vi "tkrsa6100 Config Spectrum Signal Search.vi"(0 "VISA Resource Name":refnum<visa-resource-name>, 1 "Trace (1)":enum16{"1", "2", "3", "MATH", "SGRAM"}(ring), 2 "Measurement\n(SPECTRUM)":enum16{"SPECTRUM"}(ring), 5 "Set/Read\nSearch Setting (SET)":enum16{"SET", "READ"}(ring), 7 "Search Setting\n(SEARCH ON)":T2(ring), 9 "Search Criteria\n(< THRESHOLD)":T1(ring), 11 "error in (no error)":errorcluster, 12 "Threshold (0)":dbl min=-100.0 max=10000000.0 step=1e-15 format="%#.15g", 13 "Filename\n(Empty String)":string) -> (4 "dup VISA Resource Name":refnum<visa-resource-name>, 6 "Search Setting\nResponse String":string, 8 "# Fails":i32, 15 "error out":errorcluster {"code" format="%#.0f"})   [LabVIEW 2020, in "Library Instrument & Equipement.lvlib" / "Library Spectrum Analyser.lvlib"]
doc: "Prerequisites for use:\n \nThis VI is valid in the Spectrum measurement available in the General RF Measurements group.\n\nThis VI controls the following signal search functions:\nSets/reads whether the search function is on or off\nSets/reads the trace to search\nSets/reads the search criteria\nSet/reads the search threshold\nSets/reads the status of the beep on match function\nSets/reads the status of the stop acquisitions on match function\nSets/reads the status of the autosave acquisition data on match function\nSets/reads the status of the autosave trace on match function\nSets/reads the status of the autosave picture on match function\nSaves the search mask to a file\nLoads the search mask from a file\nReads the search results\n\nerror in (no error) is checked by tkrsa6100 Write/Read wError Query.vi for any pending errors.\n\nIf error in status is ERROR:\n\nerror in (no error) and VISA Resource Name are passed straight through to error out and dup VISA Resource Name of the Write/Read Drivers and returned to the calling function. No commands are processed.\n\nIf error in status is NO ERROR:\n\nBy passing SET to Set/Read Search Setting (SET) the following parameters can be written.\nPass the following selections to enumerated control Search Setting (SEARCH ON). Additional parameters to be passed are specified with each function.\n\nOne command/query is executed per VI call.\n\nSEARCH ON\nSEARCH OFF\nEnables/disables the signal search function. No further parameters necessary to be passed.\n\nSEARCH TRACE\nSelects the trace to search. Pass the trace to enumerated control Trace (1).\n\nSEARCH CRITERIA \nSelects the criteria for the signal search. Pass the selection to enumerated control Criteria (< THRESHOLD).\n\nSEARCH THRESHOLD\nSets the threshold in dBm for the search function when the criteria is set to < Threshold or >Threshold. Pass the desired threshold to numeric control Threshold (0).\n\nNote: If this function is selected when Search Criteria is set to Inside or Outside Mask error -200 \"Execution error,Scalar operation is not currently selected\" is returned.\n\nBEEP ON MATCH ON\nBEEP ON MATCH OFF\nEnables/disables the beep on match search function. No further parameters necessary to be passed.\n\nSTOP ON MATCH ON\nSTOP ON MATCH OFF\nEnables/disables the stop acquisitions on match search function. No further parameters necessary to be passed.\n\nAUTOSAVE ACQ DATA ON MATCH ON\nAUTOSAVE ACQ DATA ON MATCH OFF\nEnables/disables the autosave acquisition data on match search function. No further parameters necessary to be passed. The file is saved to the last directory used for a Load or Save As function. The filename is <base name>-<date/time stamp>.tiq. If the base name has been changed future Save As and Autosave functions will use the new base name.\n\nAUTOSAVE TRACE ON MATCH ON\nAUTOSAVE TRACE ON MATCH OFF\nEnables/disables the autosave trace data on match search function. No further parameters necessary to be passed. The file is saved to the last directory used for a Load or Save As function. The filename is <base name>-<date/time stamp>.Specan. If the base name has been changed future Save As and Autosave functions will use the new base name.\n\nAUTOSAVE PICTURE ON MATCH ON\nAUTOSAVE PICTURE ON MATCH OFF\nEnables/disables the autosave picture on match search function. No further parameters necessary to be passed. The file is saved to the last directory used for a Load or Save As function. The filename is <base name>-<date/time stamp>.png. If the base name has been changed future Save As and Autosave functions will use the new base name.\n\nSAVE SEARCH MASK TO FILE (SET)\nSet Only\nSaves the selected search mask to a .csv file. Pass the desired file path to string control Filename (Empty String).\n\nNote: Either the filename or the full file path can be specified. No quotes are necessary around the filename and no suffix is required. The instrument firmware will add the suffix as .csv. If the full file path is not specified the file will be saved to the last directory used for Save As or Open functions. This directory can be viewed by going to the Mask Editor and selecting the Load button in the UI.\n\nLOAD SEARCH MASK FROM FILE (SET)\nSet Only\nLoads the selected search mask from a .csv file. Pass the desired file path to string control Filename (Empty String).\n\nNote: Either the filename or the full file path can be specified. No quotes are necessary around the filename and no suffix is required. The instrument firmware will add the suffix as .csv. If the full file path is not specified the file will be loaded from the last directory used for Save As or Open functions. . This directory can be viewed by going to the Mask Editor and selecting the Load button in the UI.\n\nThe following parameters can be read by passing READ to enumerated control Set/Read Search Settings (SET). Pass the following values to Search Setting (SEARCH ON). The current values are returned in string indicator Search Setting Response String.\n\nSEARCH ON\nSEARCH OFF\nEither selection returns whether the signal search function is enabled or disabled. No further parameters necessary to be passed.\n\nValid Return Values:\n0 (Disabled)\n1 (Enabled)\n\nSEARCH TRACE\nReturns the current trace that is being searched. No further parameters necessary to be passed.\n\nValid Return Values:\nSpectrum: Trace 1\nSpectrum: Trace 2\nSpectrum: Trace 3\nSpectrum: Math Trace\nSpectrum: Spectrogram Trace\n\nSEARCH CRITERIA \nReturns the criteria for the signal search. No further parameters necessary to be passed.\n\nValid Return Values:\n\nLT (Less Than Threshold)\nGT (Greater Than Threshold)\nIMAS (Inside Mask)\nOMAS (Outside Mask)\n\nSEARCH THRESHOLD\nReturns the threshold in the current vertical scale units for the search function when the criteria is set to < Threshold or >Threshold. . No further parameters necessary to be passed.\n\nValid Return Value Range: -100 to 100 (dBm)\n\nNote: The valid range is dependent on the current vertical scale units setting. \n\nBEEP ON MATCH ON\nBEEP ON MATCH OFF\nReturns whether the beep on match search function is enabled or disabled. No further parameters necessary to be passed.\n\nValid Return Values:\n0 (Disabled)\n1 (Enabled)\n\nSTOP ON MATCH ON\nSTOP ON MATCH OFF\nReturns whether the stop acquisitions on match search function is enabled or disabled. No further parameters necessary to be passed.\n\nValid Return Values:\n0 (Disabled)\n1 (Enabled)\n\nAUTOSAVE ACQ DATA ON MATCH ON\nAUTOSAVE ACQ DATA ON MATCH OFF\nReturns whether the save acquisition data on match search function is enabled or disabled. No further parameters necessary to be passed.\n\nValid Return Values:\n0 (Disabled)\n1 (Enabled)\n\nAUTOSAVE TRACE ON MATCH ON\nAUTOSAVE TRACE ON MATCH OFF\nReturns whether the save trace data on match search function is enabled or disabled. No further parameters necessary to be passed.\n\nValid Return Values:\n0 (Disabled)\n1 (Enabled)\n\nAUTOSAVE PICTURE ON MATCH ON\nAUTOSAVE PICTURE ON MATCH OFF\nReturns whether the save picture on match search function is enabled or disabled. No further parameters necessary to be passed.\n\nValid Return Values:\n0 (Disabled)\n1 (Enabled)\n\nSEARCH RESULTS (READ)\nRead Only\nReturns the results from the current signal search. No further parameters necessary to be passed.\n\nThe frequency pairs portion of the search results are returned as a comma-separated list in string indicator Search Setting Response String (see notes below). If there are no failures the frequency pairs portion will be an empty string.\n\nThe number of search violations (frequency pairs) is returned in numeric indicator # Fails. If there are no failures, a 0 will be returned.\n\nNotes on Signal Search Results\n\nAll frequencies returned are in Hz.\n\nWhen either the fixed threshold or variable frequency/amplitude search mask is used the highlighted area displayed in the UI is the area that will trigger a mask violation if a signal is present inside of it.\n\nSearch results returns the number of failures and pairs of frequencies, the first being the lowest frequency that violated the mask and the second being the frequency at which the mask violation ceased.\n\nIf the displayed signal begins outside the violation area, then enters the violation area and stays within the violation area to the maximum on-screen frequency the frequencies returned are the violation frequency and the maximum on-screen frequency.\n\nIf the displayed signal begins within the violation area and then transitions out of it, the frequencies returned are the minimum on-screen frequency and the frequency at which the violation ceased.\n\nIf the entire displayed signal is in the violation area, the frequencies returned are the lowest and highest on-screen frequencies.\n\nIf the entire displayed signal is outside the violation area, the results query returns a 0.\n\nComplete Response String Format: # failures,min violation freq1,max violation freq1;min violation freq2,max violation freq2;……min violation freq(n),max violation freq(n)\n\nThe driver separates the response string at the first comma and returns # failures as an integer in numeric indicator # Fails and the remaining frequency pairs in string indicator Search Setting Response String.\n\nThe appropriate command/query string is passed to tkrsa6100 Write/Read wError Query.vi. VI Input Error Query? is set to YES by default so query SYST:ERR? is appended to the command string and the current error information is returned in cluster Error Out. \nOn completion dup VISA Resource Name, Error Out, and Search Setting Response String are returned to the calling function."
uses:
  Library Spectrum Analyser.lvlib
panel:
  # "RSA6100 Config Spectrum Signal Search Driver"
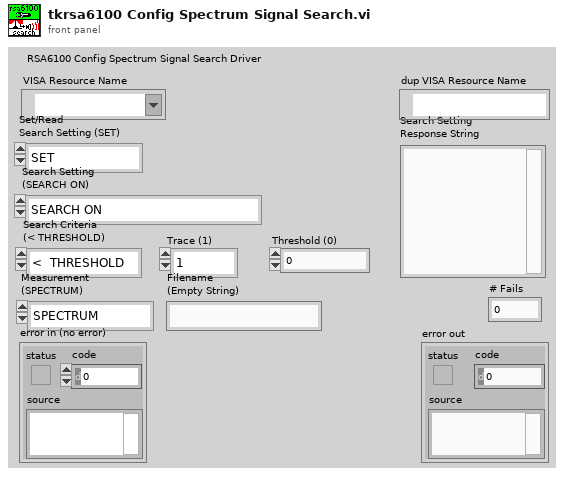
[diagram p1: front panel]
types:
  T1 = enum16{"<  THRESHOLD", "> THRESHOLD", "INSIDE MASK", "OUTSIDE MASK"}
  T2 = enum16{"SEARCH ON", "SEARCH OFF", "SEARCH TRACE", "SEARCH CRITERIA", "SEARCH THRESHOLD", "BEEP ON MATCH ON", "BEEP ON MATCH OFF", "STOP ON MATCH ON", "STOP ON MATCH OFF", "AUTOSAVE ACQ DATA ON MATCH ON", "AUTOSAVE ACQ DATA ON MATCH OFF", "AUTOSAVE TRACE ON MATCH ON", "AUTOSAVE TRACE ON MATCH OFF", "AUTOSAVE PICTURE ON MATCH ON", "AUTOSAVE PICTURE ON MATCH OFF", "SAVE SEARCH MASK TO FILE (SET)", "LOAD SEARCH MASK FROM FILE (SET)", "SEARCH RESULTS (READ)"}
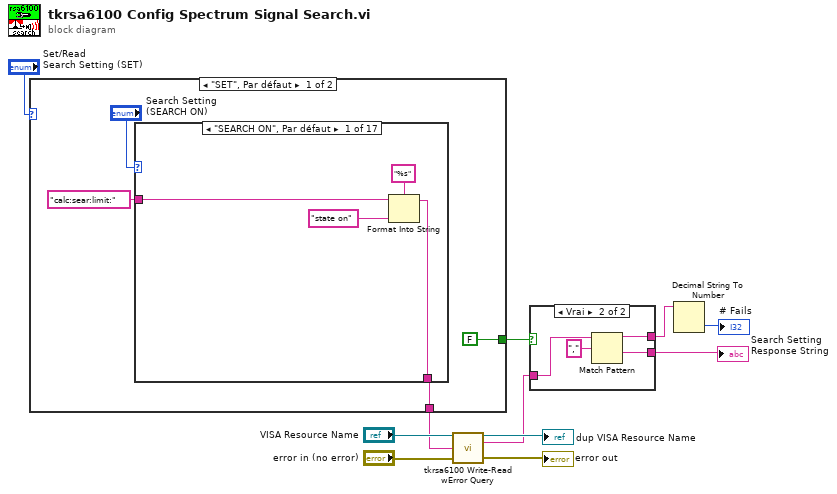
[diagram p0: block diagram]
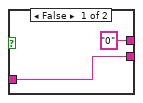
[diagram p2: hidden frame]
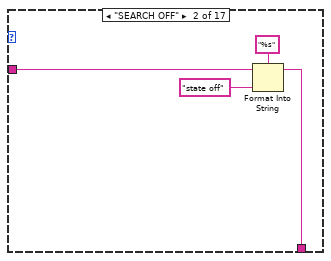
[diagram p3: hidden frame]
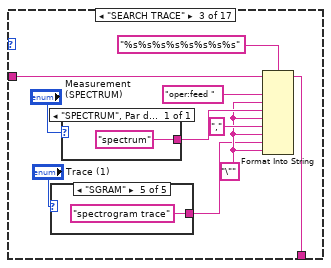
[diagram p4: hidden frame]
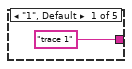
[diagram p5: hidden frame]
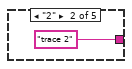
[diagram p6: hidden frame]
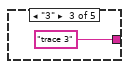
[diagram p7: hidden frame]
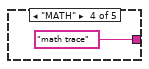
[diagram p8: hidden frame]
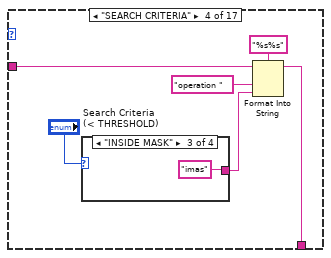
[diagram p9: hidden frame]
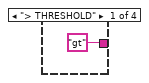
[diagram p10: hidden frame]
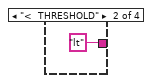
[diagram p11: hidden frame]
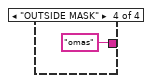
[diagram p12: hidden frame]
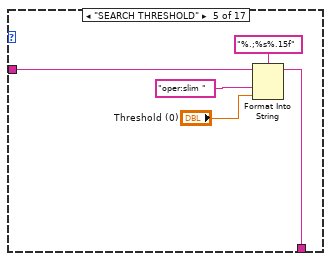
[diagram p13: hidden frame]
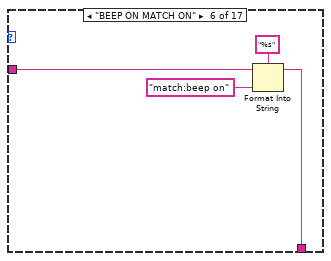
[diagram p14: hidden frame]
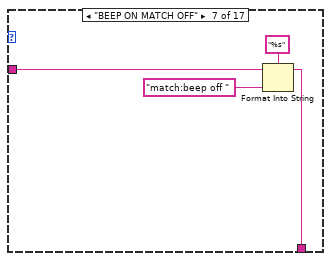
[diagram p15: hidden frame]
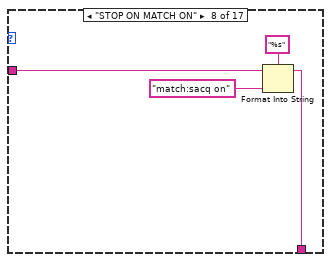
[diagram p16: hidden frame]
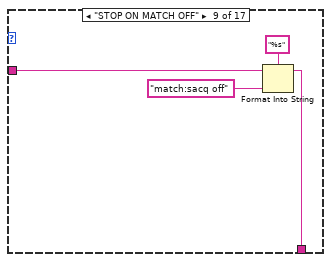
[diagram p17: hidden frame]
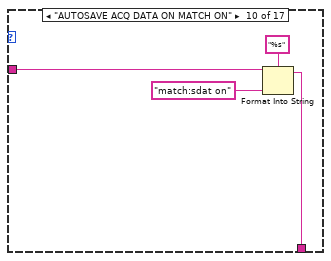
[diagram p18: hidden frame]
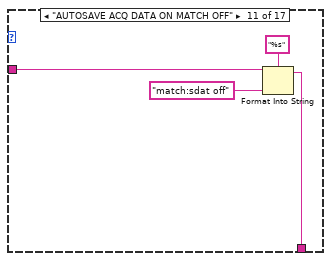
[diagram p19: hidden frame]
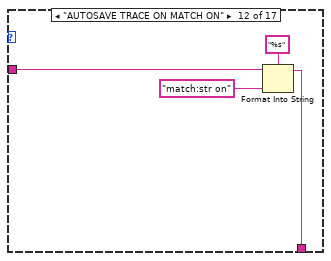
[diagram p20: hidden frame]
diagram:
  n1 = case shown="\"SET\", Par défaut" "Set/Read\nSearch Setting (SET)" {
    tunnel: [w15 w109] -> w6
    tunnel: [FALSE w107] -> w4
    frame "SET", Default {
      n2 = case shown="\"SEARCH ON\", Par défaut" "Search Setting\n(SEARCH ON)" {
        tunnel: [w18 w22 w32 w44 w53 w57 w61 w65 w69 w73 w77 w81 w85 w89 w93 w99 w105] -> w15
        tunnel: "calc:sear:limit:" ("format string") -> [w16 w21 w29 w43 w52 w56 w60 w64 w68 w71 w75 w79 w83 w87 w91 w97 w103]
        frame "SEARCH ON", Default {
          n3 = Format Into String(format string="%s", initial string=w16, "state on" ("input 1")) -> (resulting string=w18:string)  [unwired: 1 in, 1 out]
        }
        frame "SEARCH OFF" {
          n4 = Format Into String(format string="%s", initial string=w21, "state off" ("input 1")) -> (resulting string=w22:string)  [unwired: 1 in, 1 out]
        }
        frame "SEARCH TRACE" {
          w25 = "\"" ("input 1")
          n5 = case shown="\"SGRAM\"" "Trace (1)" {
            tunnel: ["trace 1" ("format string") "trace 2" ("format string") "trace 3" ("format string") "math trace" ("format string") "spectrogram trace" ("format string")] -> w24
            frame "1", Default {
            }
            frame "2" {
            }
            frame "3" {
            }
            frame "MATH" {
            }
            frame "SGRAM" {
            }
          }
          n6 = case shown="\"SPECTRUM\", Par défaut" "Measurement\n(SPECTRUM)" {
            tunnel: ["spectrum" ("format string")] -> w28
            frame "SPECTRUM", Default {
            }
          }
          n7 = Format Into String(format string="%s%s%s%s%s%s%s%s", initial string=w29, "oper:feed " ("input 1"), w25, w28, w25, "," ("input 1"), w25, w24, w25) -> (resulting string=w32:string)  [unwired: 1 in, 1 out]
        }
        frame "SEARCH CRITERIA" {
          n8 = case shown="\"INSIDE MASK\"" "Search Criteria\n(< THRESHOLD)" {
            tunnel: ["gt" ("input 1") "lt" ("input 1") "imas" ("input 1") "omas" ("input 1")] -> w40
            frame "> THRESHOLD" {
            }
            frame "<  THRESHOLD" {
            }
            frame "INSIDE MASK" {
            }
            frame "OUTSIDE MASK" {
            }
          }
          n9 = Format Into String(format string="%s%s", initial string=w43, "operation " ("input 1"), w40) -> (resulting string=w44:string)  [unwired: 1 in, 1 out]
        }
        frame "SEARCH THRESHOLD" {
          n10 = Format Into String(format string="%.;%s%.15f", initial string=w52, "oper:slim " ("input 1"), "Threshold (0)") -> (resulting string=w53:string)  [unwired: 1 in, 1 out]
        }
        frame "BEEP ON MATCH ON" {
          n11 = Format Into String(format string="%s", initial string=w56, "match:beep on" ("input 1")) -> (resulting string=w57:string)  [unwired: 1 in, 1 out]
        }
        frame "BEEP ON MATCH OFF" {
          n12 = Format Into String(format string="%s", initial string=w60, "match:beep off " ("input 1")) -> (resulting string=w61:string)  [unwired: 1 in, 1 out]
        }
        frame "STOP ON MATCH ON" {
          n13 = Format Into String(format string="%s", initial string=w64, "match:sacq on" ("input 1")) -> (resulting string=w65:string)  [unwired: 1 in, 1 out]
        }
        frame "STOP ON MATCH OFF" {
          n14 = Format Into String(format string="%s", initial string=w68, "match:sacq off" ("input 1")) -> (resulting string=w69:string)  [unwired: 1 in, 1 out]
        }
        frame "AUTOSAVE ACQ DATA ON MATCH ON" {
          n15 = Format Into String(format string="%s", initial string=w71, "match:sdat on" ("input 1")) -> (resulting string=w73:string)  [unwired: 1 in, 1 out]
        }
        frame "AUTOSAVE ACQ DATA ON MATCH OFF" {
          n16 = Format Into String(format string="%s", initial string=w75, "match:sdat off" ("input 1")) -> (resulting string=w77:string)  [unwired: 1 in, 1 out]
        }
        frame "AUTOSAVE TRACE ON MATCH ON" {
          n17 = Format Into String(format string="%s", initial string=w79, "match:str on" ("input 1")) -> (resulting string=w81:string)  [unwired: 1 in, 1 out]
        }
        frame "AUTOSAVE TRACE ON MATCH OFF" {
          n18 = Format Into String(format string="%s", initial string=w83, "match:str off" ("input 1")) -> (resulting string=w85:string)  [unwired: 1 in, 1 out]
        }
        frame "AUTOSAVE PICTURE ON MATCH ON" {
          n19 = Format Into String(format string="%s", initial string=w87, "match:spic on" ("input 1")) -> (resulting string=w89:string)  [unwired: 1 in, 1 out]
        }
        frame "AUTOSAVE PICTURE ON MATCH OFF" {
          n20 = Format Into String(format string="%s", initial string=w91, "match:spic off" ("input 1")) -> (resulting string=w93:string)  [unwired: 1 in, 1 out]
        }
        frame "SAVE SEARCH MASK TO FILE (SET)" {
          w96 = "\"" ("input 1")
          n21 = local read "Filename\n(Empty String)"() -> (w98:string)
          n22 = Format Into String(format string="%s%s%s%s", initial string=w97, "oper:mask:store " ("input 1"), w96, w98, w96) -> (resulting string=w99:string)  [unwired: 1 in, 1 out]
        }
        frame "LOAD SEARCH MASK FROM FILE (SET)" {
          w102 = "\"" ("input 1")
          n23 = Format Into String(format string="%s%s%s%s", initial string=w103, "oper:mask:load " ("input 1"), w102, "Filename\n(Empty String)", w102) -> (resulting string=w105:string)  [unwired: 1 in, 1 out]
        }
      }
    }
    frame "READ" {
      n24 = local read "Search Setting\n(SEARCH ON)"() -> (w108:T2)
      n25 = case shown="\"SEARCH RESULTS (READ)\"" w108 {
        tunnel: ["calc:sear:lim:state?" ("Command") "calc:sear:lim:state?" ("Command") "calc:sear:lim:oper:feed?" ("Command") "calc:sear:lim:oper?" ("Command") "calc:sear:lim:oper:slim?" ("Command") "calc:sear:lim:match:beep?" ("Command") "calc:sear:lim:match:beep?" ("Command") "calc:sear:lim:match:sacq?" ("Command") "calc:sear:lim:match:sacq?" ("Command") "calc:sear:lim:match:sdat?" ("Command") "calc:sear:lim:match:sdat?" ("Command") "calc:sear:lim:match:str?" ("Command") "calc:sear:lim:match:str?" ("Command") "calc:sear:lim:match:spic?" ("Command") "calc:sear:lim:match:spic?" ("Command") "calc:sear:lim:report:data?" ("Command")] -> w109
        tunnel: [FALSE FALSE FALSE FALSE FALSE FALSE FALSE FALSE FALSE FALSE FALSE FALSE FALSE FALSE FALSE TRUE] -> w107
        frame "SEARCH ON", Default {
        }
        frame "SEARCH OFF" {
        }
        frame "SEARCH TRACE" {
        }
        frame "SEARCH CRITERIA" {
        }
        frame "SEARCH THRESHOLD" {
        }
        frame "BEEP ON MATCH ON" {
        }
        frame "BEEP ON MATCH OFF" {
        }
        frame "STOP ON MATCH ON" {
        }
        frame "STOP ON MATCH OFF" {
        }
        frame "AUTOSAVE ACQ DATA ON MATCH ON" {
        }
        frame "AUTOSAVE ACQ DATA ON MATCH OFF" {
        }
        frame "AUTOSAVE TRACE ON MATCH ON" {
        }
        frame "AUTOSAVE TRACE ON MATCH OFF" {
        }
        frame "AUTOSAVE PICTURE ON MATCH ON" {
        }
        frame "AUTOSAVE PICTURE ON MATCH OFF" {
        }
        frame "SEARCH RESULTS (READ)" {
        }
      }
    }
  }
  n26 = call "tkrsa6100 Write-Read wError Query.vi"("VISA Resource Name"="VISA Resource Name", "Command (Empty String)"=w6, "error in (no error)"="error in (no error)") -> ("dup VISA Resource Name"=→"dup VISA Resource Name":refnum<visa-resource-name>, "Response"=w5:string, "error out"=→"error out":errorcluster)  [unwired: 4 in, 6 out]
  n27 = case shown="Vrai" w4 {
    tunnel: w5 -> [w143 w146]
    tunnel: ["0" ("Response") w145] -> w2
    tunnel: [w143 w144] -> w3
    frame False {
    }
    frame True {
      n28 = Match Pattern(string=w146, regular expression=",") -> (before substring=w145:string, after substring=w144:string)  [unwired: 3 out]
    }
  }
  "Search Setting\nResponse String" <- w3
  n29 = Decimal String To Number(string=w2) -> (number=→"# Fails":i32)  [unwired: 3 out]
